vi "LC_PV_React_Ctrl.vi"   [LabVIEW 2016]
doc: "-----------------------------------------------------------------------------------------------------------------------\nCopyright <2019> <The University of Tennessee at Knoxville and the University of Tennessee Research Foundation>\nThis software is released under BSD-3\nhttps://opensource.org/licenses/BSD-3-Clause \nAdditional license options available at https://utrf.tennessee.edu/industry/sample-agreements/\n-----------------------------------------------------------------------------------------------------------------------\n\n\nReactive power support for PV local controller"
uses:
  LabVIEW Data/MathScriptVIs/MCStatic_36913153632_137dbbc8b62ff179ad17ce13afb809c8.vi
  <instcachedir>/0/MCStatic_36913153632_137dbbc8b62ff179ad17ce13afb809c8_7337D6D141B744C0ACEB8CFFCA4DAD86.lvgen/MCStatic_36913153632_137dbbc8b62ff179ad17ce13afb809c8_7337D6D141B744C0ACEB8CFFCA4DAD86_001.vi
  <vilib>/imath/engines/lvmath2/RunTimeEngine/NodeEndStatement/NIMS_NodeEndStatement_Output.vi
  <instcachedir>/0/NIMS_NodeEndStatement_Output_53EC0D466D134D7ABD903AC30B43404B.lvgen/NIMS_NodeEndStatement_Output_53EC0D466D134D7ABD903AC30B43404B_001.vi
  <vilib>/imath/engines/lvmath2/RunTimeEngine/ErrorHandling/NIMS_Finalize Error.vi
  BESS_LC/PIcontroller.m
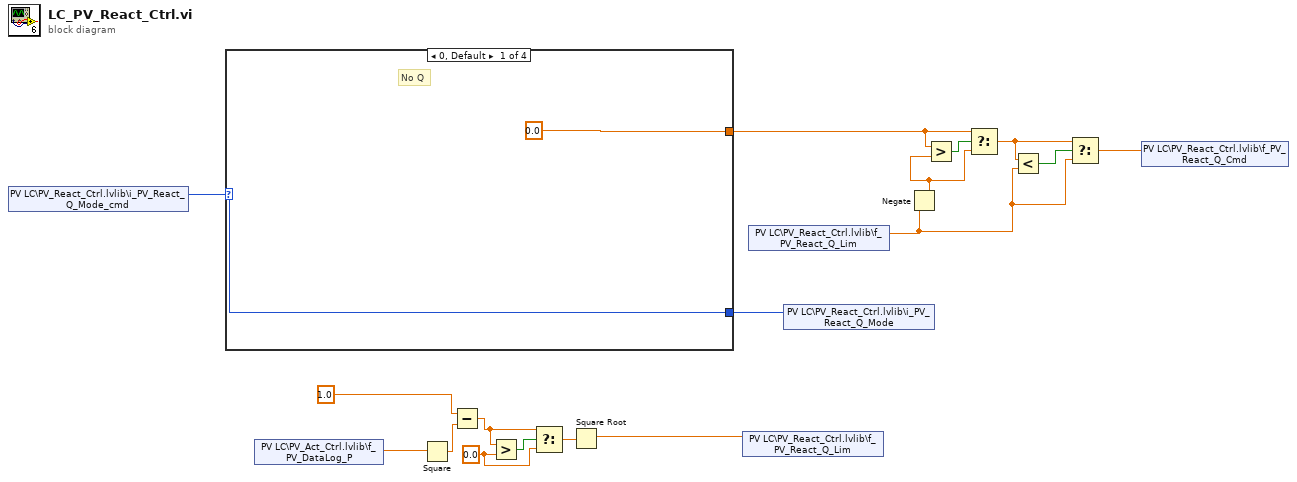
[diagram p0: block diagram]
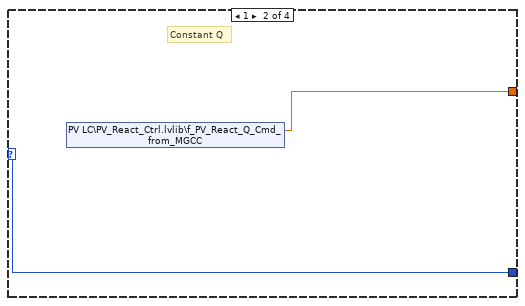
[diagram p2: hidden frame]
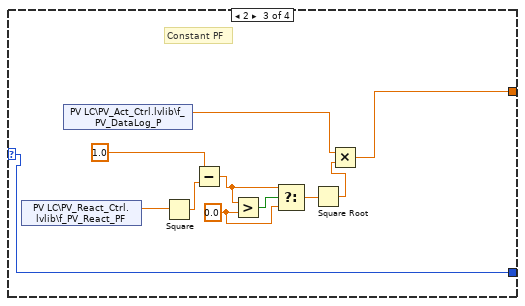
[diagram p3: hidden frame]
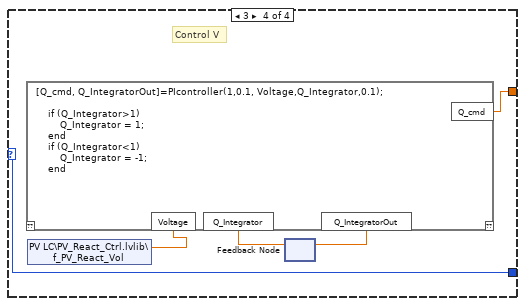
[diagram p4: hidden frame]
diagram:
  w3 = 0.0 ("y")
  n1 = shared-variable "PV LC\\PV_React_Ctrl.lvlib\\i_PV_React_Q_Mode_cmd"() -> (w17:i16)  [unwired: 1 in, 1 out]
  n2 = case shown="0, Default" w17 {
    selector: w17 -> [w18 w21 w22 w37]
    tunnel: [0.0 ("f_Batt1_React_Q_cmd") w20 w23 w36] -> w14
    tunnel: [w18 w21 w22 w37] -> w16
    frame 0, Default {
      # "No Q"
    }
    frame 1 {
      # "Constant Q"
      n3 = shared-variable "PV LC\\PV_React_Ctrl.lvlib\\f_PV_React_Q_Cmd_from_MGCC"() -> (w20:dbl)  [unwired: 1 in, 1 out]
    }
    frame 2 {
      w26 = 0.0 ("y")
      # "Constant PF"
      n4 = shared-variable "PV LC\\PV_React_Ctrl.lvlib\\f_PV_React_PF"() -> (w32:dbl)  [unwired: 1 in, 1 out]
      n5 = shared-variable "PV LC\\PV_Act_Ctrl.lvlib\\f_PV_DataLog_P"() -> (w25:dbl)  [unwired: 1 in, 1 out]
      n6 = Square(x=w32) -> (x^2=w31:dbl)
      n7 = Subtract(x=1.0 ("f_Batt1_React_Q_lim"), y=w31) -> (x-y=w27:dbl)
      n8 = Greater?(x=w27, y=w26) -> (0:w29:bool)
      n9 = Select(t=w27, s=w29, f=w26) -> (s? t:f=w28:dbl)
      n10 = Square Root(x=w28) -> (sqrt(x)=w24:dbl)
      n11 = Multiply(x=w25, y=w24) -> (x*y=w23:dbl)
    }
    frame 3 {
      # "Control V"
      n12 = shared-variable "PV LC\\PV_React_Ctrl.lvlib\\f_PV_React_Vol"() -> (w33:dbl)  [unwired: 1 in, 1 out]
      n13 = feedback #1() -> (w34:dbl)  [unwired: 1 in]
      n14 = mathscript code="[Q_cmd, Q_IntegratorOut]=PIcontroller(1,0.1, Voltage,Q_Integrator,0.1);\n   \n    if (Q_Integrator>1)\n        Q_Integrator = 1;\n    end \n    if (Q_Integrator<1)\n        Q_Integrator = -1;\n    end"("Voltage"=w33, "Q_Integrator"=w34) -> ("Q_cmd"=w36:dbl, "Q_IntegratorOut"=w35:dbl)  [unwired: 1 in, 1 out]
      n15 = feedback-in #1(w35) -> ()
    }
  }
  n16 = shared-variable "PV LC\\PV_Act_Ctrl.lvlib\\f_PV_DataLog_P"() -> (w2:dbl)  [unwired: 1 in, 1 out]
  n17 = Square(x=w2) -> (x^2=w8:dbl)
  n18 = Subtract(x=1.0 ("f_Batt1_React_Q_lim"), y=w8) -> (x-y=w4:dbl)
  n19 = Greater?(x=w4, y=w3) -> (0:w6:bool)
  n20 = Select(t=w4, s=w6, f=w3) -> (s? t:f=w5:dbl)
  n21 = Square Root(x=w5) -> (sqrt(x)=w1:dbl)
  n22 = shared-variable "PV LC\\PV_React_Ctrl.lvlib\\f_PV_React_Q_Lim"(w1) -> ()  [unwired: 1 in, 1 out]
  n23 = shared-variable "PV LC\\PV_React_Ctrl.lvlib\\f_PV_React_Q_Lim"() -> (w11:dbl)  [unwired: 1 in, 1 out]
  n24 = shared-variable "PV LC\\PV_React_Ctrl.lvlib\\i_PV_React_Q_Mode"(w16) -> ()  [unwired: 1 in, 1 out]
  n25 = Negate(x=w11) -> (-x=w13:dbl)
  n26 = Greater?(x=w14, y=w13) -> (0:w15:bool)
  n27 = Select(t=w14, s=w15, f=w13) -> (s? t:f=w12:dbl)
  n28 = Less?(x=w12, y=w11) -> (x < y?=w10:bool)
  n29 = Select(t=w12, s=w10, f=w11) -> (s? t:f=w9:dbl)
  n30 = shared-variable "PV LC\\PV_React_Ctrl.lvlib\\f_PV_React_Q_Cmd"(w9) -> ()  [unwired: 1 in, 1 out]
